vi "SPADQ_TrigDelay.vi"(6 "Delay in Pts":i32, 8 "error in (no error)":errorcluster, 9 "adq_num":i32, 10 "adq_cu_ptr in":refnum<k24>, 11 "ADQAPI Ref":refnum<k24>) -> (0 "error out":errorcluster, 2 "ADQ_SetPreTrigSamples":i32, 3 "ADQAPI Ref (out)":refnum<k24>)   [LabVIEW 2022 SP3]
doc: "_____AlazarTech, Scope_____\n\nSet the Trigger delay"
uses:
  C:/Windows/System32/ADQAPI_dotNet_helper.dll
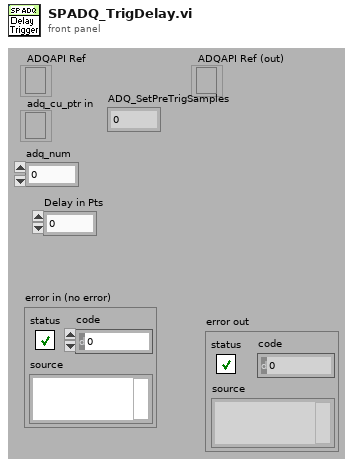
[diagram p1: front panel]
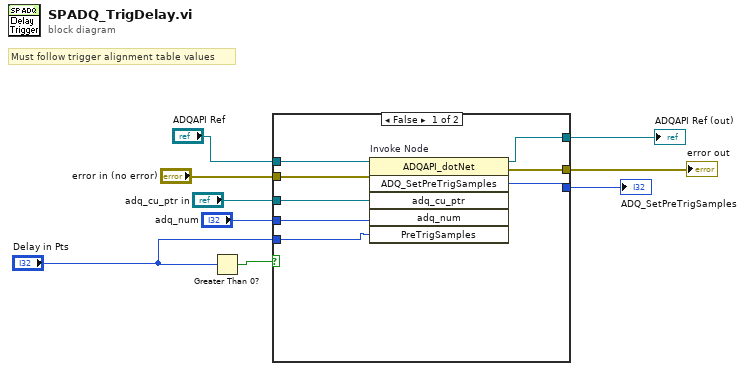
[diagram p0: block diagram]
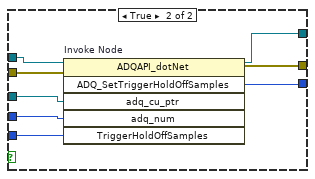
[diagram p2: hidden frame]
diagram:
  # "Must follow trigger alignment table values"
  n1 = Greater Than 0?(x="Delay in Pts") -> (x > 0?=w9:bool)
  n2 = case shown="False" w9 {
    tunnel: "error in (no error)" -> [w17 w25]
    tunnel: [w16 w24] -> w7
    tunnel: "adq_num" -> [w15 w23]
    tunnel: "Delay in Pts" -> [w14 w22]
    tunnel: "ADQAPI Ref" -> [w13 w20]
    tunnel: [w12 w21] -> w4
    tunnel: "adq_cu_ptr in" -> [w11 w19]
    tunnel: [w10 w18] -> w2
    frame False {
      n3 = invoke on="Invoke Node" class="ADQAPI_dotNet" method="ADQ_SetPreTrigSamples"(reference=w13, error in=w17, "adq_cu_ptr"=w11, "adq_num"=w15, "PreTrigSamples"=w14) -> (reference out=w12:refnum<k24>, error out=w16:errorcluster, "ADQ_SetPreTrigSamples"=w10:i32)  [unwired: 1 in, 3 out]
    }
    frame True {
      n4 = invoke on="Invoke Node" class="ADQAPI_dotNet" method="ADQ_SetTriggerHoldOffSamples"(reference=w20, error in=w25, "adq_cu_ptr"=w19, "adq_num"=w23, "TriggerHoldOffSamples"=w22) -> (reference out=w21:refnum<k24>, error out=w24:errorcluster, "ADQ_SetTriggerHoldOffSamples"=w18:i32)  [unwired: 1 in, 3 out]
    }
  }
  "error out" <- w7
  "ADQAPI Ref (out)" <- w4
  "ADQ_SetPreTrigSamples" <- w2
